vi "Serial Init IMU.vi"(6 "stop bits (10: 1 bit)":u16(ring)=10 items=["1 bit"=10, "1.5 bits"=15, "2 bits"=20], 7 "Invert Polarity?":bool, 8 "error in (no error)":errorcluster, 10 "data bits (8)":i32=8 min=5 max=8 step=1, 11 "baud rate (9600)":u32=115200) -> (0 "error out":errorcluster, 3 "FPGA IMU OUT":refnum<k20>)   [LabVIEW 2016]
uses:
  <vilib>/rvi/interface/nirviMethod/nirviMethod.xnode
  <vilib>/rvi/interface/nirviOpenFPGA/nirviOpenFPGA.xnode
  <vilib>/rvi/interface/nirviReadWriteControl/nirviReadWriteControl.xnode
  FPGA Bitfiles/FPGAIMU_FPGATarget_FPGAIMURead_c-b2E2IVPMQ.lvbitx
  <vilib>/FPGAPlugInAG/roboRIO/niLvFpga_Open_roboRIO.vi
  <vilib>/FPGAPlugInAG/roboRIO/niLvFpga_Reset_roboRIO.vi
  <vilib>/rvi/errors/niLvFpgaMergeErrorWithErrorCode.vi
  <vilib>/rvi/errors/niLvFpgaAdjustHostInterfaceError.vi
  <vilib>/FPGAPlugInAG/roboRIO/niLvFpga_Run_roboRIO.vi
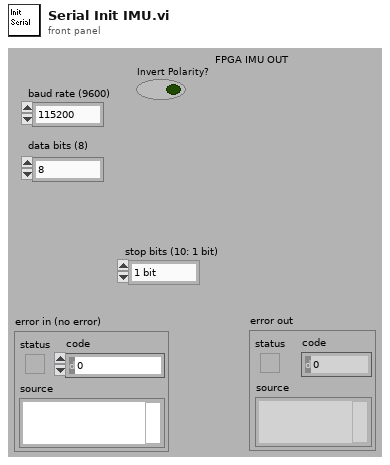
[diagram p1: front panel]
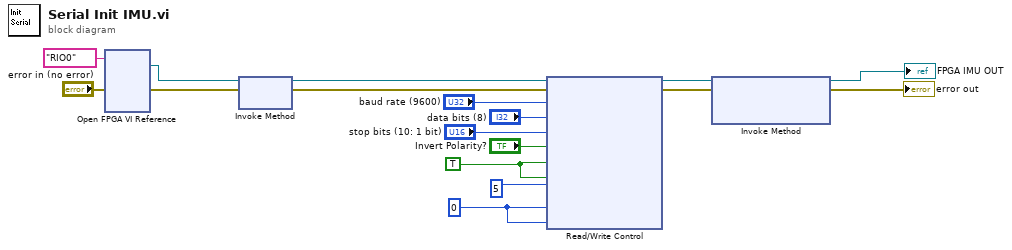
[diagram p0: block diagram]
diagram:
  w1 = u32 0 ("FirstTune")
  w4 = TRUE ("Start imu")
  n1 = xnode "Open FPGA VI Reference"("error in"="error in (no error)", "resource name"=tag "RIO0") -> ("FPGA VI Reference Out"=w14:refnum<k20>, "error out"=w13:errorcluster)
  n2 = xnode "Invoke Method"("FPGA VI Reference In"=w14, "error in"=w13) -> ("FPGA VI Reference Out"=w12:refnum<k20>, "error out"=w11:errorcluster)
  n3 = xnode "Read/Write Control"("FPGA VI Reference In"=w12, "error in"=w11, "baud rate (9600)"="baud rate (9600)", "data bits (8)"="data bits (8)", "stop bits (10: 1 bit)"="stop bits (10: 1 bit)", "Invert Polarity?"="Invert Polarity?", "Start imu"=w4, "Stop imu"=w4, "SecondTune"=u32 5 ("FirstTune"), "ThirdTune"=w1, "FirstTune"=w1) -> ("FPGA VI Reference Out"=w10:refnum<k20>, "error out"=w9:errorcluster)
  n4 = xnode "Invoke Method"("FPGA VI Reference In"=w10, "error in"=w9) -> ("FPGA VI Reference Out"=→"FPGA IMU OUT":refnum<k20>, "error out"=→"error out":errorcluster)  [unwired: 1 in]
